vi "Periodic Tasks.vi"(8 "error in":errorcluster) -> ()   [LabVIEW 2013]
doc: "This VI runs in parallel to other tasks. It can contain as many user-defined periodic loops as you need. These can carry out PID or other sorts of timed response."
uses:
  <vilib>/Rock Robotics/SystemInterfaces/Utilities/FPGA_UtilitiesLED Source.ctl
  <vilib>/Rock Robotics/SystemInterfaces/Utilities/FPGA_UtilitiesLED State.ctl
  <vilib>/Rock Robotics/WPI/Compressor/WPI_CompressorGetSetRefNum.vi
  Robot Global Data.vi
panel:
  out "Drive Loop Time":u32
  out "HandleInputElements":i32
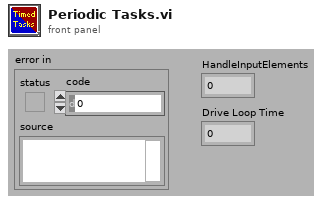
[diagram p1: front panel]
types:
  T1 = typedef "TeleopInstruction.ctl" = cluster{"cDriveLeft":dbl, "cDriveRight":dbl, "cHalfDrive":bool, "cStraightDrive":bool, "cReverseDrive":bool, "cSonicShifter":bool, "cRoller":dbl, "cCollector":dbl, "cClapper":bool, "cFiringPneumatic":bool, "cKickerPneumatic":bool, "cRollerPneumatic":bool}
  T2 = typedef "DriveQueueInstruction.ctl" = cluster{"DriveInstruction":T3, "Subsystem":T4, "Action":T5}
  T3 = typedef "DriveInstruction.ctl" = cluster{"cDriveLeft":dbl, "cDriveRight":dbl, "cHalfDrive":bool, "cStraightDrive":bool, "cReverseDrive":bool}
  T4 = typedef "QueueSubsystem.ctl" = enum16{"Drive", "SonicShifter", "Kicker", "FiringPneumatic", "Roller", "Clapper", "RollerRelay", "Collector"}
  T5 = typedef "TankDriveAction.ctl" = enum16{"Init", "LinearDrive", "SetValue", "Disable"}
  T6 = typedef "FPGA_UtilitiesLED State.ctl" = enum16{"Off", "On", "Toggle"}
  T7 = typedef "FPGA_UtilitiesLED Source.ctl" = enum16{"User LED", "FPGA LED"}
  T8 = typedef "QueueInstruction.ctl" = cluster{"Data":variant, "Subsystem":T4, "Action":T9}
  T9 = typedef "QueueAction.ctl" = enum16{"Init", "SetValue", "Disable"}
  T10 = typedef "WPI_CompressorDevRef.ctl" = cluster{"DevStatus":errorcluster, "DigitalInputDevRef":T11, "RelayDevRef":T14}
  T11 = typedef "WPI_DigitalInputDevRef.ctl" = cluster{"DevStatus":errorcluster, "DIO Channel":T12, "Digital Module":T13}
  T12 = typedef "FPGA_DIOChannel.ctl" = enum8{"DIO 1", "DIO 2", "DIO 3", "DIO 4", "DIO 5", "DIO 6", "DIO 7", "DIO 8", "DIO 9", "DIO 10", "DIO 11", "DIO 12", "DIO 13", "DIO 14", "Invalid"}
  T13 = typedef "FPGA_TypedefDigitalModule.ctl" = enum16{"Digital Module 1", "Digital Module 2"}
  T14 = typedef "WPI_RelayDevRef.ctl" = cluster{"DevStatus":errorcluster, "Relay Channel":T15, "Digital Module":T13, "Relay Direction":T16}
  T15 = typedef "FPGA_DIORelayChannel.ctl" = enum8{"Relay 1", "Relay 2", "Relay 3", "Relay 4", "Relay 5", "Relay 6", "Relay 7", "Relay 8", "Invalid"}
  T16 = typedef "WPI_RelayDirection.ctl" = enum16{"Both directions", "Forward only", "Reverse only"}
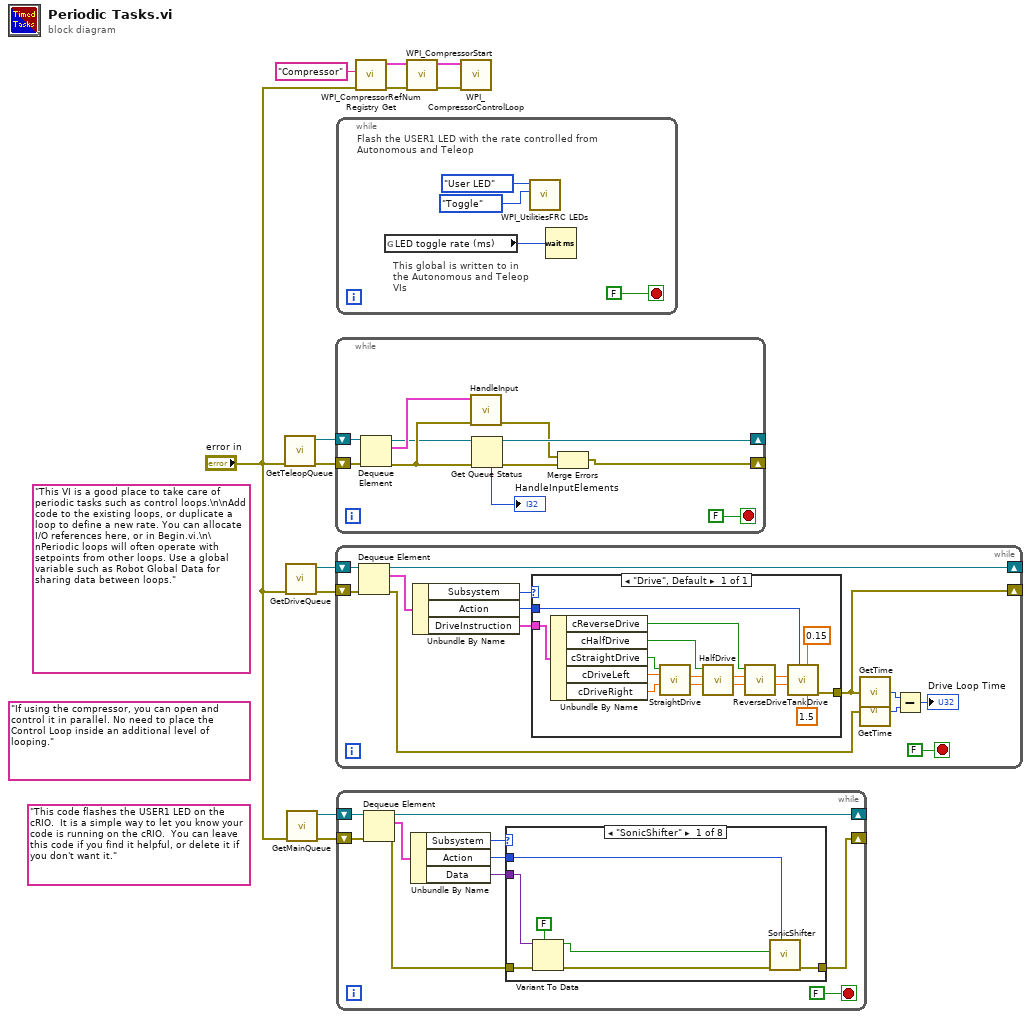
[diagram p0: block diagram]
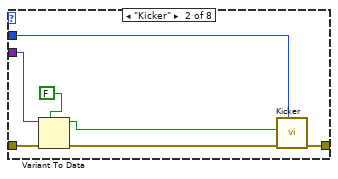
[diagram p2: hidden frame]
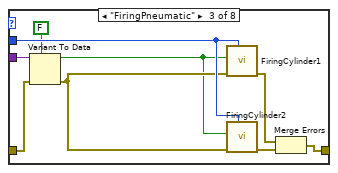
[diagram p3: hidden frame]
diagram:
  (unwired) "If using the compressor, you can open and control it in parallel. No need to place the Control Loop inside an additional level of looping."
  (unwired) "This code flashes the USER1 LED on the cRIO.  It is a simple way to let you know your code is running on the cRIO.  You can leave this code if you find it helpful, or delete it if you don't want it."
  (unwired) "This VI is a good place to take care of periodic tasks such as control loops.\n\nAdd code to the existing loops, or duplicate a loop to define a new rate. You can allocate I/O references here, or in Begin.vi.\n\nPeriodic loops will often operate with setpoints from other loops. Use a global variable such as Robot Global Data for sharing data between loops."
  n1 = call "GetTeleopQueue.vi"("error in (no error)"="error in") -> ("error out"=w6:errorcluster, "queue out"=w7:refnum<queue>)  [unwired: 9 in]
  n2 = call "GetDriveQueue.vi"("error in (no error)"="error in") -> ("error out"=w5:errorcluster, "queue out"=w4:refnum<queue>)  [unwired: 9 in]
  n3 = call "GetMainQueue.vi"("error in (no error)"="error in") -> ("error out"=w1:errorcluster, "queue out"=w2:refnum<queue>)  [unwired: 9 in]
  n4 = while {
    shift-right: [w14] -> _
    shift-left: w6 -> [w23]
    shift-right: [w21] -> _
    shift-left: w7 -> [w22]
    stop <- FALSE stop-if-true
    n5 = Dequeue Element(queue=w22, error in (no error)=w23) -> (queue out=w17:refnum<queue>, element=w19:T1, error out=w18:errorcluster)  [unwired: 1 in, 1 out]
    n6 = call "HandleInput.vi"("error in (no error)"=w18, "TeleopInstruction"=w19) -> ("error out"=w15:errorcluster)  [unwired: 9 in]
    n7 = Get Queue Status(queue=w17, error in (no error)=w18) -> (queue out=w21:refnum<queue>, error out=w16:errorcluster, # elements in queue=→"HandleInputElements":i32)  [unwired: 1 in, 5 out]
    n8 = Merge Errors(w15, w16) -> (w14:errorcluster)
  }
  n9 = while {
    shift-right: [w35] -> _
    shift-left: w4 -> [w36]
    shift-right: [w27] -> _
    shift-left: w5 -> [w34]
    stop <- FALSE stop-if-true
    n10 = Dequeue Element(queue=w36, error in (no error)=w34) -> (queue out=w35:refnum<queue>, element=w33:T2, error out=w28:errorcluster)  [unwired: 1 in, 1 out]
    n11 = Unbundle By Name(w33) -> ("Subsystem"=w32:T4, "Action"=w31:T5, "DriveInstruction"=w30:T3)
    n12 = case shown="\"Drive\", Default" w32 {
      tunnel: w31 -> [w52]
      tunnel: w30 -> [w50]
      tunnel: [w38] -> w27
      frame "Drive", Default {
        n13 = Unbundle By Name(w50) -> ("cReverseDrive"=w41:bool, "cHalfDrive"=w40:bool, "cStraightDrive"=w39:bool, "cDriveLeft"=w49:dbl, "cDriveRight"=w48:dbl)
        n14 = call "StraightDrive.vi"("RightDrive in"=w48, "LeftDrive in"=w49, "StraightDrive"=w39) -> ("RightDrive out"=w46:dbl, "LeftDrive out"=w47:dbl)  [unwired: 7 in]
        n15 = call "HalfDrive.vi"("RightDrive in"=w46, "LeftDrive in"=w47, "HalfDrive"=w40) -> ("RightDrive out"=w44:dbl, "LeftDrive out"=w45:dbl)  [unwired: 7 in]
        n16 = call "ReverseDrive.vi"("Right"=w44, "Left"=w45, "cReverseDrive"=w41) -> ("Right"=w42:dbl, "Left"=w43:dbl)  [unwired: 7 in]
        n17 = call "TankDrive.vi"("MaxMotorChange"=1.5 ("AccelRate"), "Cutoff"=0.15, "DriveAction"=w52, "RightDesired"=w42, "LeftDesired"=w43) -> ("error out"=w38:errorcluster)  [unwired: 6 in]
      }
    }
    n18 = call "GetTime.vi"("error in"=w27) -> ("Time"=w25:u32)
    n19 = call "GetTime.vi"("error in"=w28) -> ("Time"=w26:u32)
    n20 = Subtract(x=w25, y=w26) -> (x-y=→"Drive Loop Time":u32)
  }
  n21 = while {
    stop <- FALSE stop-if-true
    # "This global is written to in the Autonomous and Teleop VIs"
    # "Flash the USER1 LED with the rate controlled from Autonomous and Teleop"
    n22 = global read "Robot Global Data.vi" "LED toggle rate (ms)"() -> (w53:u32)
    n23 = call <vilib>:"WPI_UtilitiesFRC LEDs.vi"("State"=FPGA_UtilitiesLED_State."Toggle", "LED Type"=FPGA_UtilitiesLED_Source."User LED") -> ()  [unwired: 1 in, 9 out]
    n24 = Wait (ms)(milliseconds to wait=w53) -> ()  [unwired: 1 out]
  }
  n25 = while {
    shift-right: [w64] -> _
    shift-left: w2 -> [w65]
    shift-right: [w60] -> _
    shift-left: w1 -> [w66]
    stop <- FALSE stop-if-true
    n26 = Dequeue Element(queue=w65, error in (no error)=w66) -> (queue out=w64:refnum<queue>, element=w63:T8, error out=w59:errorcluster)  [unwired: 1 in, 1 out]
    n27 = Unbundle By Name(w63) -> ("Subsystem"=w61:T4, "Action"=w58:T9, "Data"=w57:variant)
    n28 = case shown="\"SonicShifter\"" w61 {
      tunnel: [w68 w80 w86 w90 w91 w92 w93 w94] -> w60
      tunnel: w59 -> [w71 w79 w83 w90 w91 w92 w93 w94]
      tunnel: w58 -> [w73 w74 w88 _ _ _ _ _]
      tunnel: w57 -> [w72 w77 w89 _ _ _ _ _]
      frame "SonicShifter" {
        n29 = Variant To Data(error in=w71, type=FALSE, Variant=w72) -> (data=w67:bool, error out=w69:errorcluster)
        n30 = call "SonicShifter.vi"("Action"=w73, "error in (no error)"=w69, "Actuate?"=w67) -> ("error out"=w68:errorcluster)  [unwired: 8 in]
      }
      frame "Kicker" {
        n31 = Variant To Data(error in=w79, type=FALSE, Variant=w77) -> (data=w75:bool, error out=w78:errorcluster)
        n32 = call "Kicker.vi"("Action"=w74, "error in (no error)"=w78, "Actuate?"=w75) -> ("error out"=w80:errorcluster)  [unwired: 8 in]
      }
      frame "FiringPneumatic" {
        n33 = Variant To Data(error in=w83, type=FALSE, Variant=w89) -> (data=w81:bool, error out=w82:errorcluster)
        n34 = call "FiringCylinder1.vi"("Action"=w88, "error in (no error)"=w82, "Actuate?"=w81) -> ("error out"=w85:errorcluster)  [unwired: 8 in]
        n35 = call "FiringCylinder2.vi"("Action"=w88, "error in (no error)"=w82, "Actuate?"=w81) -> ("error out"=w87:errorcluster)  [unwired: 8 in]
        n36 = Merge Errors(w85, w87) -> (w86:errorcluster)
      }
      frame "Roller" {
      }
      frame "Clapper" {
      }
      frame "RollerRelay" {
      }
      frame "Drive" {
        # "\"Should\" be handled in drive loop"
      }
      frame "Collector" {
      }
    }
  }
  n37 = call <vilib>:"WPI_CompressorRefNum Registry Get.vi"("error in (no error)"="error in", "refnum name"="Compressor") -> ("error out"=w11:errorcluster, "CompressorDevRef"=w10:T10)  [unwired: 8 in]
  n38 = call <vilib>:"WPI_CompressorStart.vi"("error in (no error)"=w11, "CompressorDevRef"=w10) -> ("error out"=w9:errorcluster, "CompressorDevRef"=w8:T10)  [unwired: 8 in]
  n39 = call <vilib>:"WPI_CompressorControlLoop.vi"("error in (no error)"=w9, "CompressorDevRef"=w8) -> ()  [unwired: 10 in]
